vi "GFinder.vi"   [LabVIEW 2021]
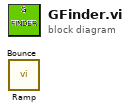
[diagram p0: block diagram]
diagram:
  n1 = call "Ramp.vi"() -> ()  [unwired: 8 in, 4 out]
  n2 = call "Bounce.vi"() -> ()  [unwired: 8 in, 4 out]
